vi "Set_Channel_Coeff_client.vi"() -> ()   [LabVIEW 2010]
doc: "This is an example of using features of the VI Server as a client. It shows how you might browse from one or more applications that may be exporting data from one or more data stations. \n\nThe example shows how to query a server for its list of exported VIs, how to get references to the VIs, and how call them with the Call By Reference function."
uses:
  Anemometry/Anemometry Sub Vis/Globals/Preference_global.vi
panel:
  in  "Set Array":T1(array[cluster]) {"Set value of D to" format="%.2f"; "Set value of C to" format="%.2f"; "Set value of B to" format="%.2f"; "Set value of A to" format="%.2f"}
  in  "server type":refnum<vi>
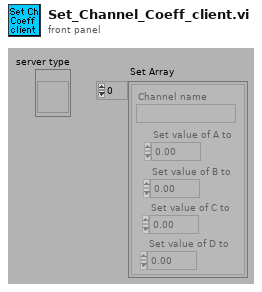
[diagram p1: front panel]
types:
  T1 = cluster{"Channel name":string, "Set value of A to":dbl, "Set value of B to":dbl, "Set value of C to":dbl, "Set value of D to":dbl}[]
  T2 = typedef "Server_Comms.ctl" = enum16{"Server Link Healthy", "Do Not Link To Server"}
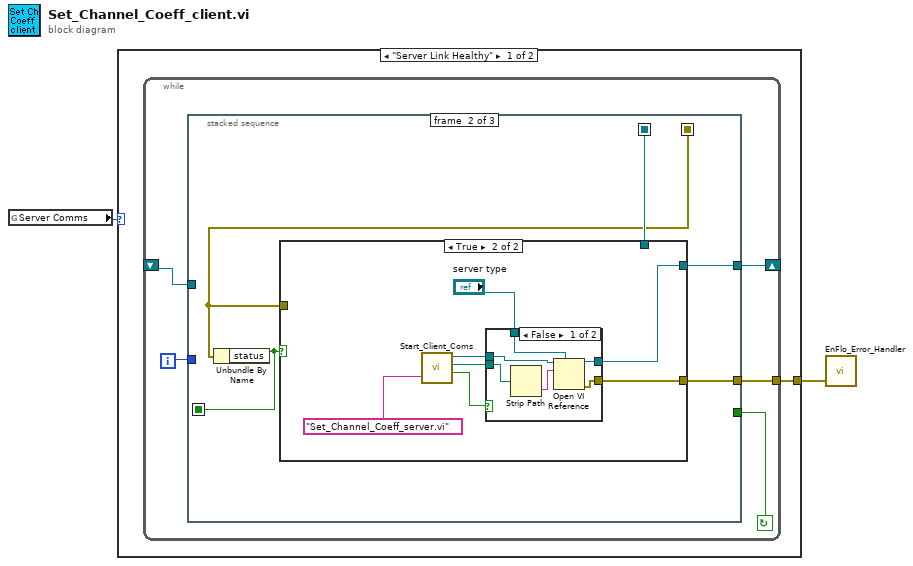
[diagram p0: block diagram]
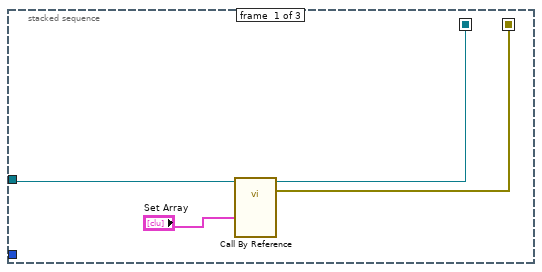
[diagram p2: hidden frame]
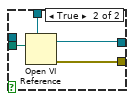
[diagram p4: hidden frame]
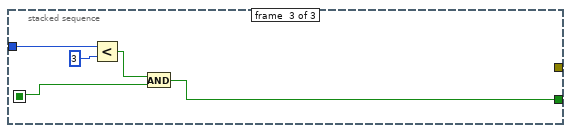
[diagram p5: hidden frame]
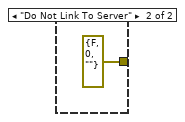
[diagram p6: hidden frame]
diagram:
  n1 = global read "Preference_global.vi" "Server Comms"() -> (w2:T2)
  n2 = case shown="\"Server Link Healthy\"" w2 {
    tunnel: [w3 errorcluster {"status"=FALSE, "code"=0, "source"=""}] -> w1
    frame "Server Link Healthy" {
      n3 = while {
        tunnel: [w4] -> w3
        shift-left: _ -> [w8]
        shift-right: [w7] -> _
        i -> [w6]
        stop <- w5 continue-if-true
        n4 = stacked-sequence {
          seq-local: [w10 _ _] -> [_ w16 _]
          seq-local: [w11 _ _] -> [_ w13 _]
          seq-local: [_ w15 _] -> [_ _ w38]
          tunnel: w8 -> [w9 _ _]
          tunnel: [_ w17 _] -> w7
          tunnel: w6 -> [_ _ w39]
          tunnel: [_ _ w37] -> w5
          tunnel: [_ w14 _] -> w4
          frame #0 {
            n5 = call-by-ref "?"(reference=w9, "Set Array"="Set Array") -> (reference out=w10:refnum<vi>, error out=w11:errorcluster)  [unwired: 1 in]
          }
          frame #1 {
            n6 = Unbundle By Name(w13) -> ("status"=w15:bool)
            n7 = case shown="True" w15 {
              tunnel: [w19 w22] -> w17
              tunnel: w16 -> [w19 _]
              tunnel: [w18 w20] -> w14
              tunnel: w13 -> [w18 _]
              frame False {
              }
              frame True {
                n8 = call "Start_Client_Coms.vi"("VI name to run on server"="Set_Channel_Coeff_server.vi") -> ("LabVIEW application reference"=w24:refnum<vi>, "Checked VI name"=w25:path, "Local Call"=w23:bool)  [unwired: 1 in, 1 out]
                n9 = case shown="False" w23 {
                  tunnel: [w31 w36] -> w22
                  tunnel: "server type" -> [w29 w35]
                  tunnel: w25 -> [w28 w34]
                  tunnel: w24 -> [w27 _]
                  tunnel: [w30 w33] -> w20
                  frame False {
                    n10 = Strip Path(path=w28) -> (name=w32:string)  [unwired: 1 out]
                    n11 = Open VI Reference(type specifier VI Refnum (for type only)=w29, application reference (local)=w27, vi path=w32) -> (vi reference=w31:refnum<vi>, error out=w30:errorcluster)  [unwired: 1 in, 2 out]
                  }
                  frame True {
                    n12 = Open VI Reference(type specifier VI Refnum (for type only)=w35, vi path=w34) -> (vi reference=w36:refnum<vi>, error out=w33:errorcluster)  [unwired: 1 in, 3 out]
                  }
                }
              }
            }
          }
          frame #2 {
            n13 = Less?(x=w39, y=3) -> (x < y?=w41:bool)
            n14 = And(x=w41, y=w38) -> (x .and. y?=w37:bool)
          }
        }
      }
    }
    frame "Do Not Link To Server" {
    }
  }
  n15 = call "EnFlo_Error_Handler.vi"("error in (no error)"=w1) -> ()  [unwired: 2 in, 3 out]
